vi "Register to Discovery Service.vi"(0 "gRPC ID":T2, 5 "PortNumber":i32, 7 "MeasurementPluginService in":refnum<class "Measurement Plugin Service.lvclass">, 9 "IMeasurementService in":refnum<class "IMeasurementService.lvclass">[](array[class]), 11 "error in":errorcluster) -> (4 "gRPC ID out":T2, 6 "Response Data":T1, 8 "MeasurementPluginService out":refnum<class "Measurement Plugin Service.lvclass">, 10 "IMeasurementService out":refnum<class "IMeasurementService.lvclass">[](array[class]), 15 "error out":errorcluster)   [LabVIEW 2020, in "MeasurementLink Measurement Server.lvlib"]
uses:
  MeasurementLink Measurement Server.lvlib
  MeasurementLink Discovery Client/MeasurementLink Discovery Client.lvlib
  MeasurementLink Discovery Client/RPC Messages/ni_measurementlink_discovery_v1_RegisterServiceRequest.ctl
  MeasurementLink Discovery Client/RPC Messages/ni_measurementlink_discovery_v1_ServiceLocation.ctl
  MeasurementLink Discovery Client/RPC Messages/ni_measurementlink_discovery_v1_ServiceDescriptor.ctl
  Measurement Plugin Service/Measurement Plugin Service.lvclass
  Classes/IMeasurementService/IMeasurementService.lvclass
  MeasurementLink Discovery Client/RPC Messages/ni_measurementlink_discovery_v1_ServiceDescriptor_AnnotationsEntry.ctl
  <vilib>/gRPC/LabVIEW gRPC Library/Shared/grpcId.ctl
  <vilib>/gRPC/LabVIEW gRPC Library/grpc-lvsupport-release.lvlib
  MeasurementLink Discovery Client/RPC Messages/ni_measurementlink_discovery_v1_RegisterServiceResponse.ctl
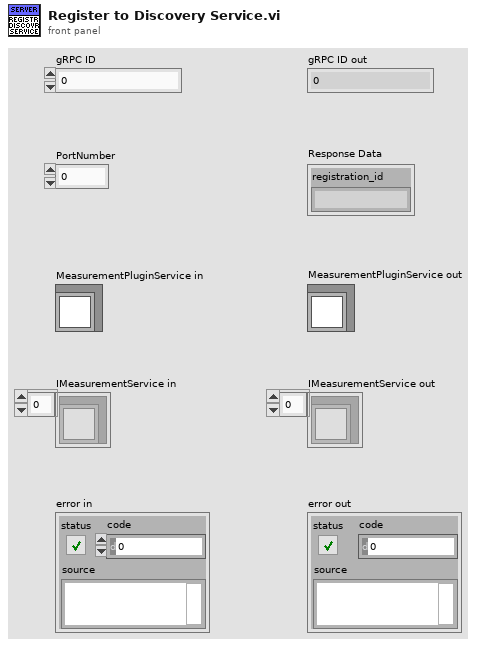
[diagram p1: front panel]
types:
  T1 = typedef "MeasurementLink Discovery Client.lvlib/ni_measurementlink_discovery_v1_RegisterServiceResponse.ctl" = cluster{"registration_id":string}
  T2 = typedef "grpc-lvsupport-release.lvlib/grpcId.ctl" = u64
  T3 = typedef "MeasurementLink Discovery Client.lvlib/ni_measurementlink_discovery_v1_RegisterServiceRequest.ctl" = cluster{"service_description":T4, "location":T6}
  T4 = typedef "MeasurementLink Discovery Client.lvlib/ni_measurementlink_discovery_v1_ServiceDescriptor.ctl" = cluster{"display_name":string, "description_url":string, "provided_interfaces":string[], "service_class":string, "annotations":T5[]}
  T5 = typedef "MeasurementLink Discovery Client.lvlib/ni_measurementlink_discovery_v1_ServiceDescriptor_AnnotationsEntry.ctl" = cluster{"key":string, "value":string}
  T6 = typedef "MeasurementLink Discovery Client.lvlib/ni_measurementlink_discovery_v1_ServiceLocation.ctl" = cluster{"location":string, "insecure_port":string, "ssl_authenticated_port":string}
  T7 = typedef "MeasurementLink Measurement Server.lvlib/MeasurementDetails.ctl" = cluster{"display_name":string, "version":string}
  T8 = typedef "MeasurementLink Measurement Server.lvlib/MeasurementAnnotation.ctl" = cluster{"key":string, "value":string}
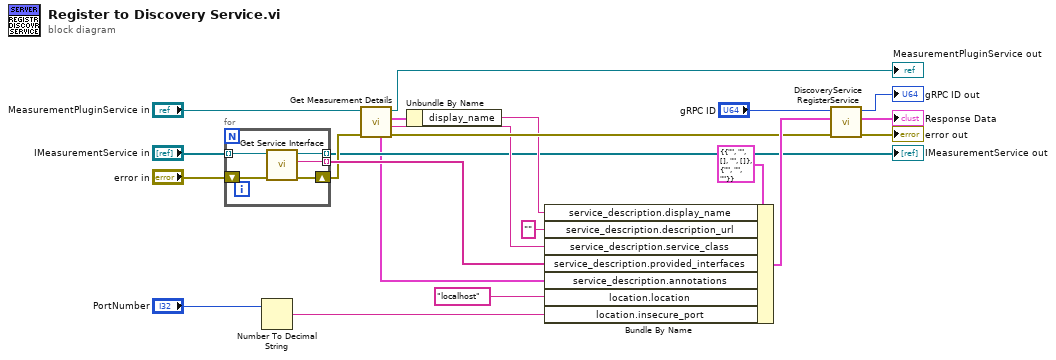
[diagram p0: block diagram]
diagram:
  n1 = for {
    tunnel: "IMeasurementService in" -> [w27] mode=indexing
    tunnel: [w26] -> w7 mode=indexing
    shift-right: [w24] -> w5
    shift-left: "error in" -> [w25]
    tunnel: [w23] -> w3 mode=indexing
    n2 = call-dynamic "Get Service Interface.vi"("error in (no error)"=w25, "IMeasurementService in"=w27) -> ("error out"=w24:errorcluster, "service interface"=w26:string, "IMeasurementService out"=w23:refnum<class "IMeasurementService.lvclass">)  [unwired: 7 in]
  }
  "IMeasurementService out" <- w3
  n3 = Number To Decimal String(number="PortNumber") -> (decimal integer string=w22:string)  [unwired: 1 in]
  n4 = call-dynamic "Get Measurement Details.vi"("error in"=w5, "MeasurementPluginService in"="MeasurementPluginService in") -> ("error out"=w11:errorcluster, "Service Class"=w9:string, "Measurement Details"=w10:T7, "MeasurementPluginService out"=→"MeasurementPluginService out":refnum<class "Measurement Plugin Service.lvclass">, "Measurement Annotations"=w1:T8[])  [unwired: 5 in]
  n5 = Unbundle By Name(w10) -> ("display_name"=w8:string)
  n6 = Bundle By Name(cluster=T3 {"service_description"={"display_name"="", "description_url"="", "provided_interfaces"=[], "service_class"="", "annotations"=[]}, "location"={"location"="", "insecure_port"="", "ssl_authenticated_port"=""}} ("Request Data"), "service_description.display_name"=w8, "service_description.description_url"="", "service_description.service_class"=w9, "service_description.provided_interfaces"=w7, "service_description.annotations"=w1, "location.location"="localhost", "location.insecure_port"=w22) -> (w17:T3)
  n7 = call "DiscoveryService RegisterService.vi"("error in"=w11, "Request Data"=w17, "gRPC ID"="gRPC ID") -> ("error out"=→"error out":errorcluster, "Response Data"=→"Response Data":T1, "gRPC ID out"=→"gRPC ID out":T2)  [unwired: 6 in]
